vi "Traces Display Multiple Plots.vi"(8 "Error In":errorcluster, 9 "Channel List":T1, 11 "Graphs In":refnum<vi>[](array[refnum])) -> (0 "Error Out":errorcluster, 3 "Graphs Out":refnum<vi>[](array[refnum]))   [LabVIEW 2019]
uses:
  Channel List.ctl
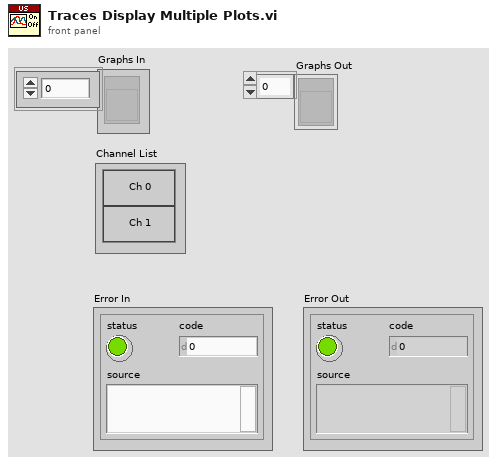
[diagram p1: front panel]
types:
  T1 = typedef "Channel List.ctl" = cluster{"Channel 0":bool, "Channel 1":bool}
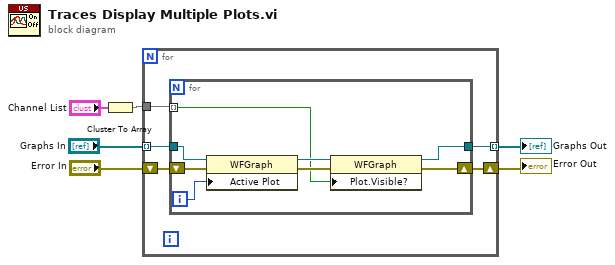
[diagram p0: block diagram]
diagram:
  n1 = Cluster To Array(cluster="Channel List") -> (array=w2:bool[])
  n2 = for {
    tunnel: w2 -> [w8]
    shift-right: [w11] -> w6
    shift-left: "Error In" -> [w10]
    tunnel: "Graphs In" -> [w7] mode=indexing
    tunnel: [w9] -> w4 mode=indexing
    n3 = for {
      shift-right: [w15] -> w11
      shift-left: w10 -> [w19]
      tunnel: w7 -> [w12]
      tunnel: [w14] -> w9
      tunnel: w8 -> [w13] mode=indexing
      i -> [w18]
      n4 = property class="WFGraph"(reference=w12, error in=w19, "Active Plot"=w18) -> (reference out=w16:refnum<vi>, error out=w17:errorcluster)
      n5 = property on="Property Node" class="WFGraph"(reference=w16, error in=w17, "Plot.Visible?"=w13) -> (reference out=w14:refnum<vi>, error out=w15:errorcluster)
    }
  }
  "Error Out" <- w6
  "Graphs Out" <- w4
